vi "Create URL.vi"(8 "error in (no error)":errorcluster, 10 "Base URL":string, 11 "URL Parameters":T1[](array[typedef])) -> (0 "error out":errorcluster, 3 "Full URL":string)   [LabVIEW 2011, in "i3-oauth.lvlib"]
doc: "Use this template to build a VI to use as a subVI."
uses:
  i3-oauth.lvlib
  Controls/key-value-pairs.ctl
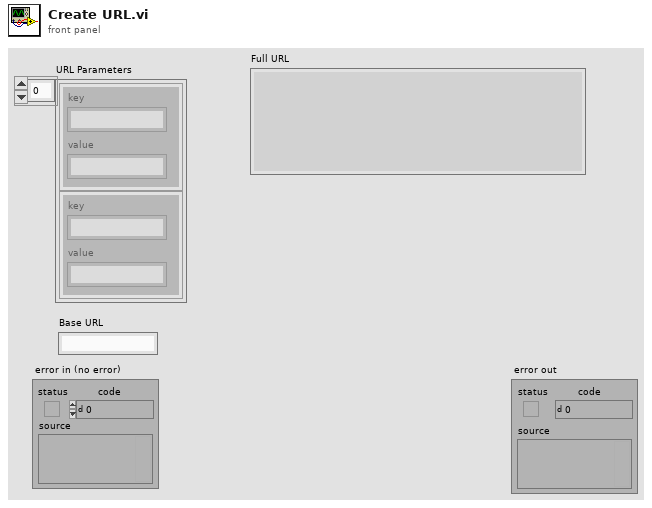
[diagram p1: front panel]
types:
  T1 = typedef "i3-oauth.lvlib/key-value-pairs.ctl" = cluster{"key":string, "value":string}
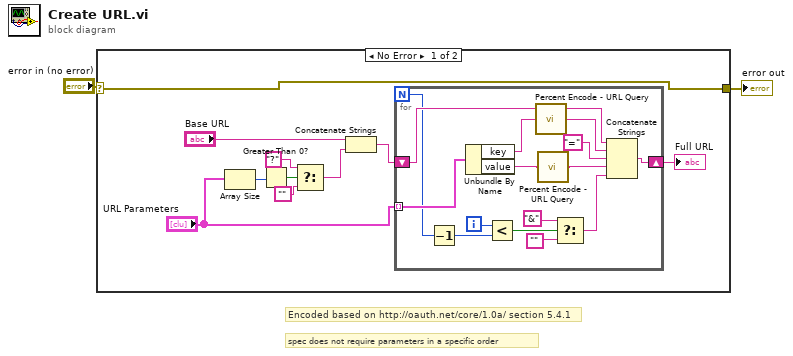
[diagram p0: block diagram]
diagram:
  # "spec does not require parameters in a specific order"
  # "Encoded based on http://oauth.net/core/1.0a/ section 5.4.1"
  n1 = case shown="No Error" "error in (no error)" {
    selector: "error in (no error)" -> [w10 w28]
    tunnel: [w10 w28] -> w1
    frame No Error {
      n2 = Array Size(array="URL Parameters") -> (size(s)=w7:i32)
      n3 = Greater Than 0?(x=w7) -> (x > 0?=w6:bool)
      n4 = Select(t="?" ("string"), s=w6, f="") -> (s? t:f=w5:string)
      n5 = Concatenate Strings("Base URL", w5) -> (w9:string)
      n6 = for {
        N -> [w22]
        shift-right: [w24] -> w12
        shift-left: w9 -> [w26]
        tunnel: "URL Parameters" -> [w27] mode=indexing
        i -> [w23]
        n7 = Decrement(x=w22) -> (x-1=w21:i32)
        n8 = Unbundle By Name(w27) -> ("key"=w17:string, "value"=w14:string)
        n9 = Less?(x=w23, y=w21) -> (x < y?=w20:bool)
        n10 = call "Percent Encode - URL Query.vi"("unescaped string in"=w17) -> ("escaped string out"=w16:string)
        n11 = call "Percent Encode - URL Query.vi"("unescaped string in"=w14) -> ("escaped string out"=w15:string)
        n12 = Select(t="&", s=w20, f="") -> (s? t:f=w13:string)
        n13 = Concatenate Strings(w26, w16, "=" ("string"), w15, w13) -> (w24:string)
      }
      "Full URL" <- w12
    }
    frame Error {
    }
  }
  "error out" <- w1
